vi "시리얼통신(11.26).vi"() -> ()   [LabVIEW 2018]
uses:
  <vilib>/Instr/_visa.llb/VISA Configure Serial Port (Instr).vi
panel:
  out "Brake":dbl
  out "시리얼 쓰기 오류":dbl
  out "시리얼 읽기 오류":dbl
  out "byte(20)":i32
  out "AorM":u8
  out "시리얼 읽기":string
  out "BATT":dbl
  out "SPEED(RPM)":i16
  out "ALIVE":u8
  out "BRAKE":u8
  out "STEER":i16
  out "GEAR":u8
  out "ESTOP":u8
  out "ETX":string
  out "ENC":string
  in  "End Program":bool
  out "error out":errorcluster
  in  "baud rate (115200)":u32=115200 min=115200 max=115200
  in  "VISA PortName":refnum<visa-resource-name>
  # "읽기"
  # "0: manual, 1: auto"
  # "0: off, 1: on"
  # "0: forward, 1: neutral, 2: backward"
  # "-150~150"
  # "-2000~2000"
  # "0~100"
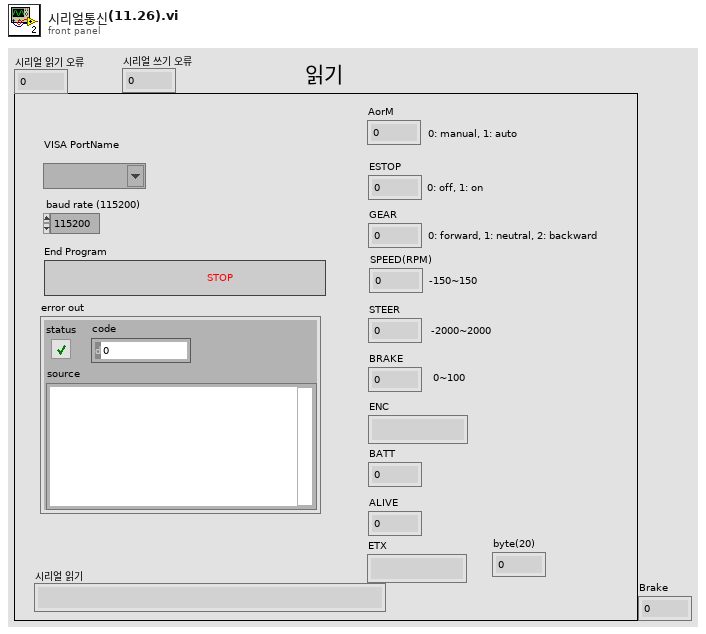
[diagram p1: front panel]
types:
  T1 = cluster{"S":u8, "T":u8, "X":u8, "AorM":u8, "E-STOP":u8, "GEAR":u8, "SPEED":u16, "STEER":i16, "BRAKE":u8, "ALIVE":u8, "ETX0":u8, "ETX1":u8}
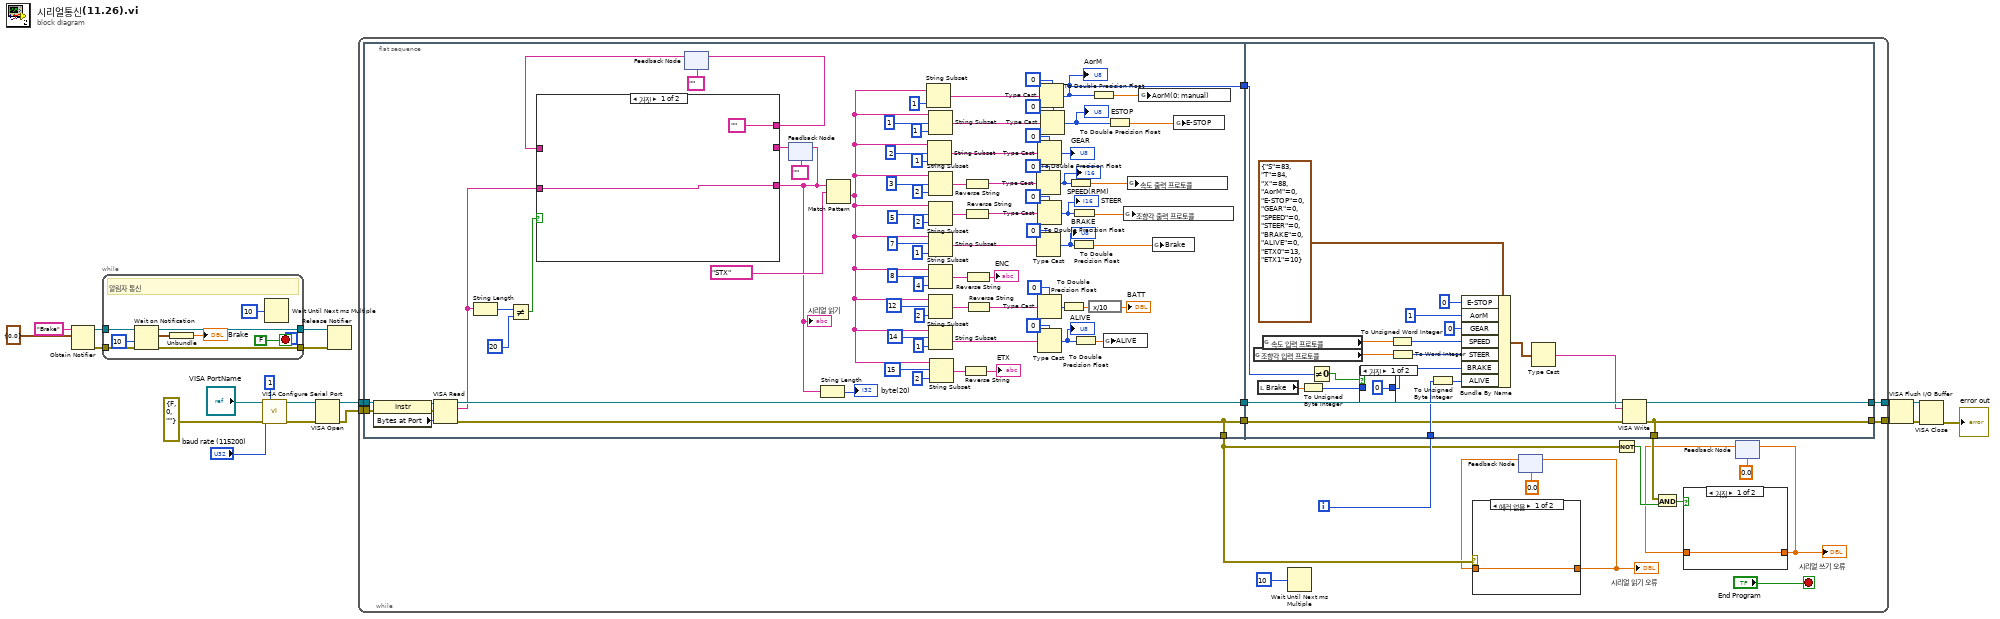
[diagram p0: block diagram]
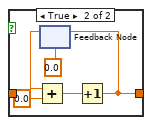
[diagram p2: hidden frame]
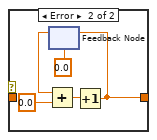
[diagram p3: hidden frame]
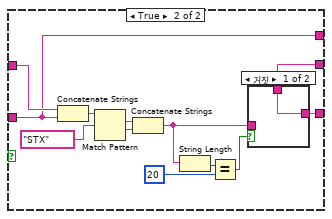
[diagram p4: hidden frame]
diagram:
  n1 = Obtain Notifier(name (unnamed)="Brake" ("이름(이름없음)"), notification data type=cluster{dbl} {0.0}) -> (notifier out=w4:refnum<notifier>, error out=w3:errorcluster)  [unwired: 2 in, 1 out]
  n2 = while {
    tunnel: w4 -> [w26]
    tunnel: w3 -> [w25]
    tunnel: [w24] -> w2
    tunnel: [w23] -> w1
    stop <- FALSE stop-if-true
    # "알림자 통신"
    n3 = Wait on Notification(notifier=w26, timeout in ms (-1)=10 ("타임아웃(ms) (-1)"), error in (no error)=w25) -> (notifier out=w24:refnum<notifier>, notification=w22:cluster{dbl}, error out=w23:errorcluster)  [unwired: 1 in, 1 out]
    n4 = Unbundle(w22) -> (→"Brake":dbl)
    n5 = Wait Until Next ms Multiple(millisecond multiple=u32 10 ("ms 배수")) -> ()  [unwired: 1 out]
  }
  n6 = call-poly "VISA Configure Serial Port"("VISA resource name"="VISA PortName", "timeout (10sec)"=u32 1, "baud rate (9600)"="baud rate (115200)", "error in (no error)"=errorcluster {"status"=FALSE, "code"=0, "source"=""}) -> ("VISA resource name out"=w15:refnum<visa-resource-name>, "error out"=w16:errorcluster)  [unwired: 10 in]
  n7 = VISA Open(error in (no error)=w16, VISA resource name=w15) -> (VISA resource name=w13:refnum<visa-resource-name>, error out=w12:errorcluster)  [unwired: 3 in]
  n8 = Release Notifier(notifier=w2, error in (no error)=w1) -> ()  [unwired: 1 in, 3 out]
  n9 = while {
    tunnel: w13 -> [w48]
    tunnel: w12 -> [w47]
    tunnel: [w42] -> w10
    tunnel: [w44] -> w9
    i -> [w41]
    stop <- "End Program" stop-if-true
    n10 = flat-sequence {
      tunnel: w48 -> [w138]
      tunnel: w47 -> [w137]
      tunnel: [w133] -> w46
      tunnel: [w64] -> w45
      tunnel: [w64] -> w36
      tunnel: [w61] -> w29
      tunnel: w46 -> [w175]
      tunnel: w45 -> [w165]
      tunnel: [w161] -> w44
      tunnel: [w162] -> w42
      tunnel: w41 -> [w170]
      tunnel: [w161] -> w38
      tunnel: w29 -> [w155]
      frame #0 {
        n11 = property class="Instr"(reference=w138, error in=w137) -> (reference out=w136:refnum<visa-resource-name>, error out=w134:errorcluster, "Bytes at Port"=w135:u32)
        n12 = VISA Read(VISA resource name=w136, byte count=w135, error in (no error)=w134) -> (VISA resource name out=w133:refnum<visa-resource-name>, read buffer=w77:string, error out=w64:errorcluster)  [unwired: 1 out]
        n13 = String Length(string=w77) -> (length=w119:i32)
        n14 = Not Equal?(x=w119, y=20) -> (x != y?=w78:bool)
        n15 = feedback #1("" ("regular expression")) -> (w75:string)
        n16 = feedback #2("" ("regular expression")) -> (w73:string)
        n17 = case shown="거짓" w78 {
          tunnel: [w140 w142] -> w71
          tunnel: w77 -> [w140 w151]
          tunnel: ["" ("regular expression") w151] -> w76
          tunnel: w75 -> [_ w152]
          tunnel: w73 -> [_ w141]
          frame False {
          }
          frame True {
            n18 = Concatenate Strings(w152, w151) -> (w150:string)
            n19 = Match Pattern(string=w150, regular expression="STX") -> (match substring=w148:string, after substring=w147:string)  [unwired: 1 in, 2 out]
            n20 = Concatenate Strings(w148, w147) -> (w143:string)
            n21 = String Length(string=w143) -> (length=w145:i32)
            n22 = Equal?(x=w145, y=20) -> (x = y?=w144:bool)
            n23 = case shown="거짓" w144 {
              tunnel: w143 -> [_ w154]
              tunnel: [w153 w154] -> w142
              tunnel: w141 -> [w153 _]
              frame False {
              }
              frame True {
              }
            }
          }
        }
        "시리얼 읽기" <- w71
        n24 = feedback-in #1(w76) -> ()
        n25 = feedback-in #2(w71) -> ()
        n26 = String Length(string=w71) -> (length=→"byte(20)":i32)
        n27 = Match Pattern(string=w71, regular expression="STX") -> (after substring=w91:string)  [unwired: 1 in, 3 out]
        n28 = String Subset(string=w91, length (rest)=1 ("길이(나머지)")) -> (substring=w88:string)  [unwired: 1 in]
        n29 = String Subset(string=w91, offset (0)=2 ("오프셋(0)"), length (rest)=1 ("길이(나머지)")) -> (substring=w86:string)
        n30 = String Subset(string=w91, offset (0)=1 ("오프셋(0)"), length (rest)=1 ("길이(나머지)")) -> (substring=w87:string)
        n31 = String Subset(string=w91, offset (0)=3 ("오프셋(0)"), length (rest)=2 ("길이(나머지)")) -> (substring=w102:string)
        n32 = String Subset(string=w91, offset (0)=5 ("오프셋(0)"), length (rest)=2 ("길이(나머지)")) -> (substring=w101:string)
        n33 = String Subset(string=w91, offset (0)=7 ("오프셋(0)"), length (rest)=1 ("길이(나머지)")) -> (substring=w83:string)
        n34 = String Subset(string=w91, offset (0)=8 ("오프셋(0)"), length (rest)=4 ("길이(나머지)")) -> (substring=w98:string)
        n35 = String Subset(string=w91, offset (0)=12 ("오프셋(0)"), length (rest)=2 ("길이(나머지)")) -> (substring=w95:string)
        n36 = String Subset(string=w91, offset (0)=14 ("오프셋(0)"), length (rest)=1 ("길이(나머지)")) -> (substring=w80:string)
        n37 = String Subset(string=w91, offset (0)=15 ("오프셋(0)"), length (rest)=2 ("길이(나머지)")) -> (substring=w92:string)
        n38 = Reverse String(1:w92) -> (0:→"ETX":string)
        n39 = Reverse String(1:w102) -> (0:w85:string)
        n40 = Reverse String(1:w101) -> (0:w84:string)
        n41 = Reverse String(1:w98) -> (0:→"ENC":string)
        n42 = Reverse String(1:w95) -> (0:w81:string)
        n43 = Type Cast(type=i16 0, x=w85) -> (*(type *) &x=w128:i16)
        "SPEED(RPM)" <- w128
        n44 = Type Cast(type=u8 0, x=w83) -> (*(type *) &x=w63:u8)
        "BRAKE" <- w63
        n45 = Type Cast(type=u8 0, x=w86) -> (*(type *) &x=→"GEAR":u8)
        n46 = Type Cast(type=i16 0, x=w84) -> (*(type *) &x=w129:i16)
        "STEER" <- w129
        n47 = Type Cast(type=u16 0, x=w81) -> (*(type *) &x=w131:u16)
        n48 = Type Cast(type=u8 0, x=w80) -> (*(type *) &x=w117:u8)
        "ALIVE" <- w117
        n49 = Type Cast(type=u8 0 ("AorM"), x=w88) -> (*(type *) &x=w61:u8)
        "AorM" <- w61
        n50 = Type Cast(type=u8 0, x=w87) -> (*(type *) &x=w66:u8)
        "ESTOP" <- w66
        n51 = To Double Precision Float(number=w131) -> (double precision float=w132:dbl)
        n52 = To Double Precision Float(number=w128) -> (double precision float=w68:dbl)
        n53 = To Double Precision Float(number=w63) -> (double precision float=w62:dbl)
        n54 = To Double Precision Float(number=w129) -> (double precision float=w69:dbl)
        n55 = To Double Precision Float(number=w117) -> (double precision float=w116:dbl)
        n56 = expression code="x/10"(w132) -> (→"BATT":dbl)
        n57 = To Double Precision Float(number=w61) -> (double precision float=w67:dbl)
        n58 = global write "글로벌 (11.25).vi" "ALIVE"(w116) -> ()
        n59 = To Double Precision Float(number=w66) -> (double precision float=w65:dbl)
        n60 = global write "글로벌 (11.25).vi" "조향각 출력 프로토콜"(w69) -> ()
        n61 = global write "글로벌 (11.25).vi" "속도 출력 프로토콜"(w68) -> ()
        n62 = global write "글로벌 (11.25).vi" "AorM(0: manual)"(w67) -> ()
        n63 = global write "글로벌 (11.25).vi" "Brake"(w62) -> ()
        n64 = global write "글로벌 (11.25).vi" "E-STOP"(w65) -> ()
      }
      frame #1 {
        n65 = global read "글로벌 (11.25).vi" "조향각 입력 프로토콜"() -> (w166:dbl)
        n66 = local read "Brake"() -> (w159:dbl)
        n67 = global read "글로벌 (11.25).vi" "속도 입력 프로토콜"() -> (w167:dbl)
        n68 = To Unsigned Byte Integer(number=w159) -> (unsigned 8bit integer=w158:u8)
        n69 = Not Equal To 0?(x=w155) -> (x != 0?=w156:bool)
        n70 = case shown="거짓" w156 {
          tunnel: w158 -> [_ w177]
          tunnel: [u8 0 w177] -> w157
          frame False {
          }
          frame True {
          }
        }
        n71 = To Unsigned Word Integer(number=w167) -> (unsigned 16bit integer=w169:u16)
        n72 = To Word Integer(number=w166) -> (16bit integer=w168:i16)
        n73 = To Unsigned Byte Integer(number=w170) -> (unsigned 8bit integer=w171:u8)
        n74 = Bundle By Name(cluster=T1 {"S"=83, "T"=84, "X"=88, "AorM"=0, "E-STOP"=0, "GEAR"=0, "SPEED"=0, "STEER"=0, "BRAKE"=0, "ALIVE"=0, "ETX0"=13, "ETX1"=10}, "E-STOP"=u8 0, "AorM"=u8 1 ("E-STOP"), "GEAR"=u8 0, "SPEED"=w169, "STEER"=w168, "BRAKE"=w157, "ALIVE"=w171) -> (w173:T1)
        n75 = Type Cast(x=w173) -> (*(type *) &x=w172:string)  [unwired: 1 in]
        n76 = VISA Write(VISA resource name=w175, write buffer=w172, error in (no error)=w165) -> (VISA resource name out=w162:refnum<visa-resource-name>, error out=w161:errorcluster)  [unwired: 1 out]
      }
    }
    n77 = Wait Until Next ms Multiple(millisecond multiple=u32 10 ("대기 시간 (ms)")) -> ()  [unwired: 1 out]
    n78 = feedback #3(0.0) -> (w34:dbl)
    n79 = case shown="에러 없음" w36 {
      tunnel: [w55 w56] -> w35
      tunnel: w34 -> [w55 _]
      frame No Error {
      }
      frame Error {
        n80 = feedback #4(0.0) -> (w60:dbl)
        n81 = Add(x=w60, y=0.0) -> (x+y=w57:dbl)
        n82 = Increment(x=w57) -> (x+1=w56:dbl)
        n83 = feedback-in #4(w56) -> ()
      }
    }
    "시리얼 읽기 오류" <- w35
    n84 = feedback-in #3(w35) -> ()
    n85 = Not(x=w36) -> (.not. x?=w39:bool)
    n86 = And(x=w38, y=w39) -> (x .and. y?=w37:bool)
    n87 = feedback #5(0.0) -> (w31:dbl)
    n88 = case shown="거짓" w37 {
      tunnel: [w49 w50] -> w32
      tunnel: w31 -> [w49 _]
      frame False {
      }
      frame True {
        n89 = feedback #6(0.0) -> (w53:dbl)
        n90 = Add(x=w53, y=0.0) -> (x+y=w51:dbl)
        n91 = Increment(x=w51) -> (x+1=w50:dbl)
        n92 = feedback-in #6(w50) -> ()
      }
    }
    "시리얼 쓰기 오류" <- w32
    n93 = feedback-in #5(w32) -> ()
  }
  n94 = VISA Flush I/O Buffer(VISA resource name=w10, error in (no error)=w9) -> (VISA resource name out=w8:refnum<visa-resource-name>, error out=w7:errorcluster)  [unwired: 1 in]
  n95 = VISA Close(VISA resource name=w8, error in (no error)=w7) -> (error out=→"error out":errorcluster)
